vi "startConsoleUi.vi"(8 "error in (no error)":errorcluster, 11 "Handler.UserEvent.Console in":refnum<class "Handler.UserEvent.Console.lvclass">) -> (0 "error out":errorcluster, 3 "Handler.UserEvent.Console out":refnum<class "Handler.UserEvent.Console.lvclass">)   [LabVIEW 2017, in "Error Log.lvlib" / "Handler.UserEvent.Console.lvclass"]
uses:
  Handler.UserEvent.Console.lvclass
  Handler.UserEvent.Console.lvclass/Handler.UserEvent.Console.ctl
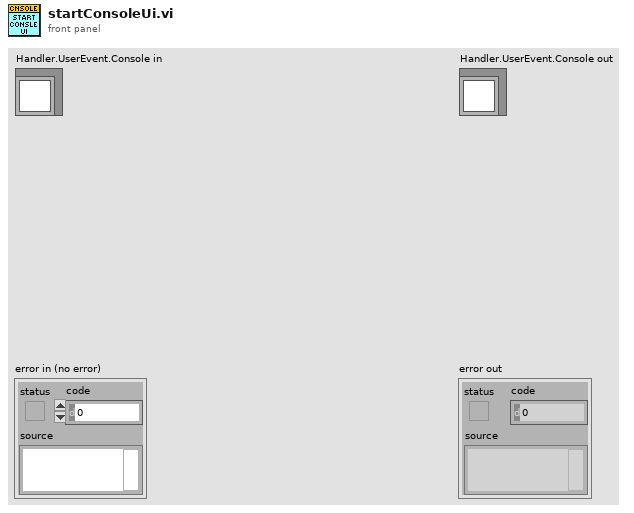
[diagram p1: front panel]
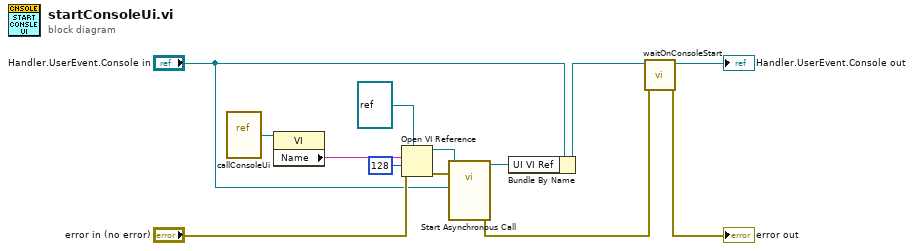
[diagram p0: block diagram]
diagram:
  n1 = vi-ref "callConsoleUi.vi"() -> (w13:refnum<vi>)
  n2 = property class="VI"(reference=w13) -> ("Name"=w12:string)  [unwired: 1 in, 2 out]
  n3 = Open VI Reference(type specifier VI Refnum (for type only)=refnum<vi> refnum, vi path=w12, options=128, error in (no error)="error in (no error)") -> (vi reference=w11:refnum<vi>, error out=w8:errorcluster)  [unwired: 2 in]
  n4 = call-by-ref "Start Asynchronous Call"(reference=w11, error in=w8, "Handler.UserEvent.Console in"="Handler.UserEvent.Console in") -> (reference out=w5:refnum<vi>, error out=w2:errorcluster)  [unwired: 9 in, 2 out]
  n5 = Bundle By Name(cluster="Handler.UserEvent.Console in", "UI VI Ref"=w5) -> (w4:refnum<class "Handler.UserEvent.Console.lvclass">)
  n6 = call "waitOnConsoleStart.vi"("error in (no error)"=w2, "Handler.UserEvent.Console in"=w4) -> ("error out"=→"error out":errorcluster, "Handler.UserEvent.Console out"=→"Handler.UserEvent.Console out":refnum<class "Handler.UserEvent.Console.lvclass">)  [unwired: 8 in]
